vi "Init_Ring.vi"(1 "Elements available":T1(array[cluster])) -> (0 "Array":cluster{"string":string, i32}[](array[cluster]))   [LabVIEW 2009]
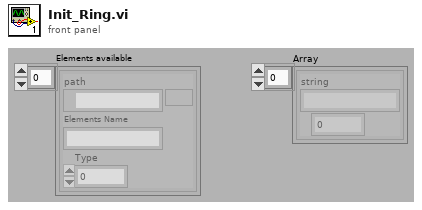
[diagram p1: front panel]
types:
  T1 = cluster{"path":path, "Elements Name":string, "Type":i32}[]
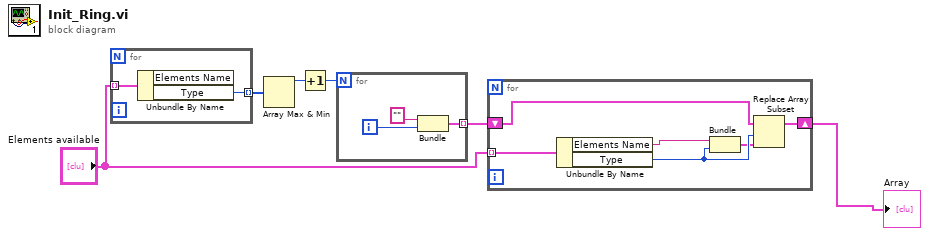
[diagram p0: block diagram]
diagram:
  n1 = for {
    tunnel: "Elements available" -> [w8] mode=indexing
    tunnel: [w7] -> w4 mode=indexing
    n2 = Unbundle By Name(w8) -> ("Type"=w7:i32)  [unwired: 1 out]
  }
  n3 = Array Max & Min(array=w4) -> (max value=w3:i32)  [unwired: 3 out]
  n4 = Increment(x=w3) -> (x+1=w2:i32)
  n5 = for {
    N: w2 -> [_]
    tunnel: [w10] -> w6 mode=indexing
    i -> [w9]
    n6 = Bundle("String"="", w9) -> (w10:cluster{"String":string, i32})  [unwired: 1 in]
  }
  n7 = for {
    tunnel: "Elements available" -> [w17] mode=indexing
    shift-right: [w13] -> w1
    shift-left: w6 -> [w16]
    n8 = Unbundle By Name(w17) -> ("Elements Name"=w12:string, "Type"=w15:i32)
    n9 = Bundle("Elements Name"=w12, "Type"=w15) -> (w14:cluster{"Elements Name":string, "Type":i32})  [unwired: 1 in]
    n10 = Replace Array Subset(array=w16, new element=w14, index=w15) -> (w13:cluster{"String":string, i32}[])
  }
  "Array" <- w1
